vi "Get Cell.vi"(8 "error in":errorcluster, 10 "Cell Address":string="A", 11 "Row in":refnum<k24>) -> (0 "error out":errorcluster, 2 "Cell":refnum<k24>, 3 "Row out":refnum<k24>)   [LabVIEW 2019, in "Open Xml.lvlib"]
doc: "Returns Cell with specified address if existing."
uses:
  Open Xml.lvlib
  D:/git/Open-Xml-LabVIEW/Source/DocumentFormat.OpenXml.dll
  DocumentFormat.OpenXml.dll
  D:/git/Open-Xml-LabVIEW/Source/DocumentFormat.OpenXml.Framework.dll
  DocumentFormat.OpenXml.Framework.dll
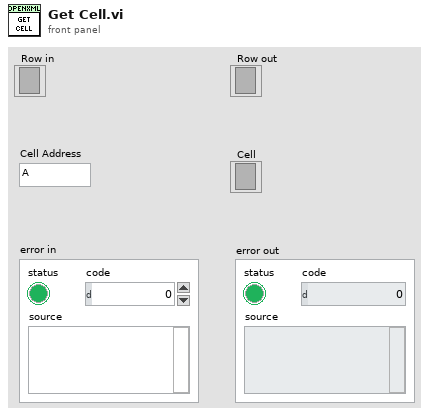
[diagram p1: front panel]
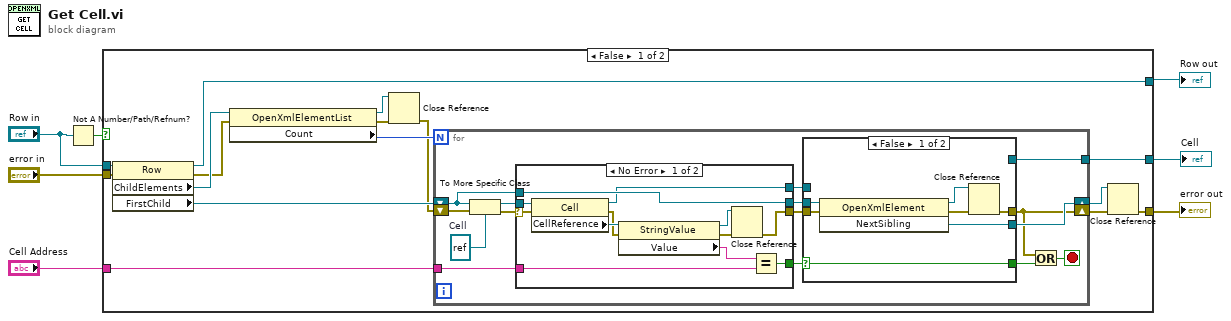
[diagram p0: block diagram]
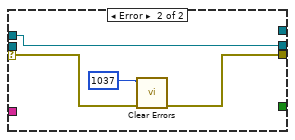
[diagram p2: hidden frame]
diagram:
  n1 = Not A Number/Path/Refnum?(number/path/refnum="Row in") -> (NaN/Path/Refnum?=w2:bool)
  n2 = case shown="False" w2 {
    tunnel: "error in" -> [w13 w65]
    tunnel: "Row in" -> [w12 w64]
    tunnel: "Cell Address" -> [w11 _]
    tunnel: [w10 w64] -> w5
    tunnel: [w9 w65] -> w4
    tunnel: [w8 _] -> w3
    frame False {
      n3 = property class="Row"(reference=w12, error in=w13) -> (reference out=w10:refnum<k24>, error out=w14:errorcluster, "ChildElements"=w22:refnum<k24>, "FirstChild"=w20:refnum<k24>)
      n4 = property class="OpenXmlElementList"(reference=w22, error in=w14) -> (reference out=w17:refnum<k24>, error out=w16:errorcluster, "Count"=w21:i32)
      n5 = Close Reference(reference=w17, error in (no error)=w16) -> (error out=w15:errorcluster)
      n6 = for {
        N: w21 -> [_]
        shift-right: [w28] -> w18
        shift-left: w20 -> [w34]
        tunnel: w11 -> [w32]
        tunnel: [w24] -> w8
        shift-right: [w27] -> w19
        shift-left: w15 -> [w36]
        stop <- w31 stop-if-true
        w37 = refnum<k24> refnum  # Cell
        n7 = To More Specific Class(target class=w37, reference=w34, error in=w36) -> (specific class reference=w33:refnum<k24>, error out=w35:errorcluster)
        n8 = case shown="No Error" w35 {
          selector: w35 -> [w49 w53]
          tunnel: [w38 w51] -> w30
          tunnel: w34 -> [w43 w52]
          tunnel: [w43 w52] -> w29
          tunnel: [w44 _] -> w23
          tunnel: w33 -> [w48 _]
          tunnel: w32 -> [w45 _]
          tunnel: [w42 _] -> w25
          frame No Error {
            n9 = property class="Cell"(reference=w48, error in=w49) -> (reference out=w42:refnum<k24>, error out=w41:errorcluster, "CellReference"=w47:refnum<k24>)
            n10 = property class="StringValue"(reference=w47, error in=w41) -> (reference out=w39:refnum<k24>, error out=w40:errorcluster, "Value"=w46:string)
            n11 = Close Reference(reference=w39, error in (no error)=w40) -> (error out=w38:errorcluster)
            n12 = Equal?(x=w46, y=w45) -> (x = y?=w44:bool)
          }
          frame Error {
            n13 = call <vilib>:"Clear Errors.vi"("error in (no error)"=w53, "specific error code to clear (0: all)"=1037) -> ("error out"=w51:errorcluster)  [unwired: 4 in, 1 out]
          }
        }
        n14 = case shown="False" w23 {
          selector: w23 -> [w54 w63]
          tunnel: w30 -> [w60 w62]
          tunnel: w29 -> [w58 _]
          tunnel: [w57 _] -> w28
          tunnel: [w55 w62] -> w27
          tunnel: [w54 w63] -> w26
          tunnel: w25 -> [_ w61]
          tunnel: [_ w61] -> w24
          frame False {
            n15 = invoke class="OpenXmlElement" method="NextSibling"(reference=w58, error in=w60) -> (reference out=w56:refnum<k24>, error out=w59:errorcluster, "NextSibling"=w57:refnum<k24>)  [unwired: 1 in]
            n16 = Close Reference(reference=w56, error in (no error)=w59) -> (error out=w55:errorcluster)
          }
          frame True {
          }
        }
        n17 = Or(x=w27, y=w26) -> (x .or. y?=w31:bool)
      }
      n18 = Close Reference(reference=w18, error in (no error)=w19) -> (error out=w9:errorcluster)
    }
    frame True {
    }
  }
  "error out" <- w4
  "Row out" <- w5
  "Cell" <- w3
